vi "Read Raw Bus Monitor Log.vi"(5 "Component ID":u8, 7 "FPGA Interface":refnum<class "FPGA Interface.lvclass">, 8 "error in (no error)":errorcluster, 11 "Bus Monitor in":refnum<class "Bus Monitor.lvclass">) -> (0 "error out":errorcluster, 1 "Raw Bus B Monitor Log":u16[](array[numeric]), 2 "Raw Bus A Monitor Log":u16[](array[numeric]), 3 "Bus Monitor out":refnum<class "Bus Monitor.lvclass">)   [LabVIEW 2016, in "BCI-1553 API.lvlib" / "Bus Monitor.lvclass"]
doc: "Read the current log stored by the bus monitor for both Bus A and Bus B. Depending on the data rates int he system, these logs may roll-over at various times in the application execution. This outputs only the raw 16-bit words stored in the bus monitor memory. The data is organized as such:\n\nIndex 0: Block Status\nIndex 1-3: Timestamp\nIndex 4: CMD1\nIndex 5: CMD2\nIndex 6: STS1\nIndex 7: STS2\nIndex 8: Word Count\nIndex 9+: Data Words\n\nThis pattern will continue until all items are accounted for or the allotted memory space has been fully used."
uses:
  Bus Monitor.lvclass
  Dependencies/FPGA Interface/FPGA Interface.lvclass
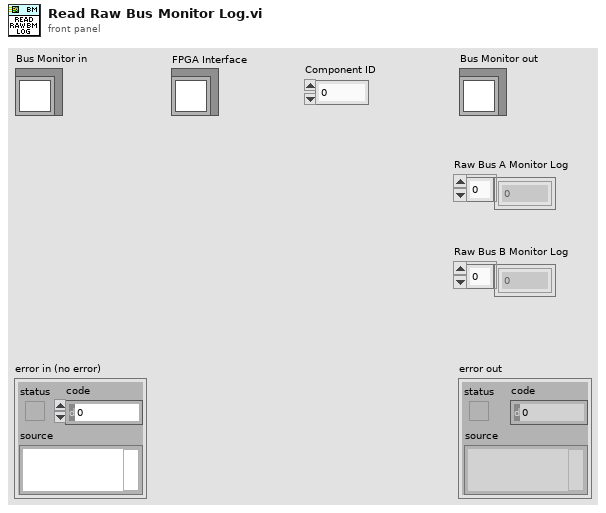
[diagram p1: front panel]
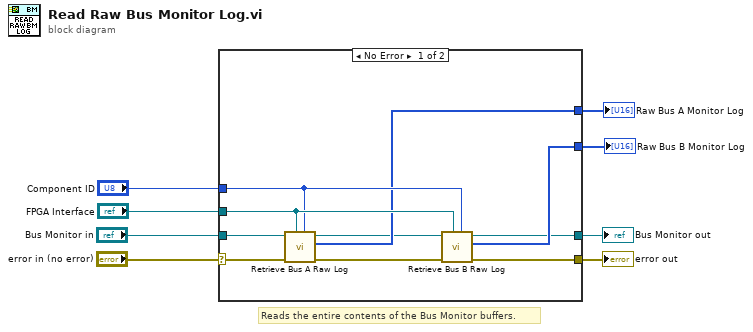
[diagram p0: block diagram]
diagram:
  # "Reads the entire contents of the Bus Monitor buffers."
  n1 = case shown="No Error" "error in (no error)" {
    selector: "error in (no error)" -> [w17 w20]
    tunnel: [w10 w20] -> w7
    tunnel: [w9 w19] -> w5
    tunnel: "Bus Monitor in" -> [w18 w19]
    tunnel: "FPGA Interface" -> [w16 _]
    tunnel: "Component ID" -> [w15 _]
    tunnel: [w14 _] -> w2
    tunnel: [w13 _] -> w1
    frame No Error {
      n2 = call "Retrieve Bus A Raw Log.vi"("Component ID"=w15, "FPGA Interface"=w16, "error in (no error)"=w17, "Bus Monitor in"=w18) -> ("error out"=w11:errorcluster, "Bus A Raw Log"=w14:u16[], "Bus Monitor out"=w12:refnum<class "Bus Monitor.lvclass">)  [unwired: 5 in]
      n3 = call "Retrieve Bus B Raw Log.vi"("Component ID"=w15, "FPGA Interface"=w16, "error in (no error)"=w11, "Bus Monitor in"=w12) -> ("error out"=w10:errorcluster, "Bus A Raw Log"=w13:u16[], "Bus Monitor out"=w9:refnum<class "Bus Monitor.lvclass">)  [unwired: 5 in]
    }
    frame Error {
    }
  }
  "error out" <- w7
  "Bus Monitor out" <- w5
  "Raw Bus A Monitor Log" <- w2
  "Raw Bus B Monitor Log" <- w1
